vi "equations.vi"() -> ()   [LabVIEW 2018]
panel:
  in  "b":dbl
  out "y2":dbl
  in  "m":dbl
  out "y1":dbl
  in  "X variable":dbl
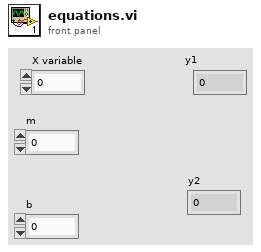
[diagram p1: front panel]
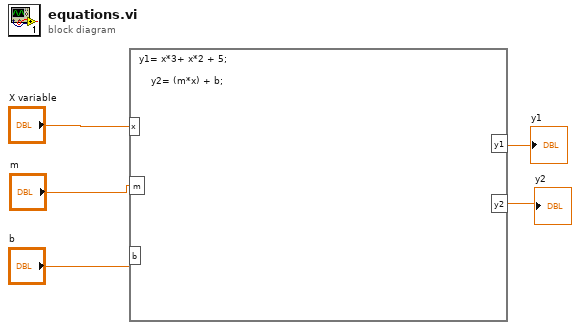
[diagram p0: block diagram]
diagram:
  n1 = formula code="y1= x*3+ x*2 + 5;\n   \n    y2= (m*x) + b;"("x"="X variable", "m"="m", "b"="b") -> ("y1"=→"y1":dbl, "y2"=→"y2":dbl)
